vi "Digital Read Pin.vi"(8 "Error In":errorcluster, 10 "Digital I/O Pin (2)":u8=2, 11 "ChipKit Resource":T1={"COM Port"="", "Board Type"=enum."ChipKit uC32", "Connection Type"=enum."USB / Serial", "Baud Rate (115200)"=15, "Bytes Per Packet (15)"=15}) -> (0 "Error Out":errorcluster, 2 "Value":bool, 3 "ChipKit Resource":T1={"COM Port"="", "Board Type"=enum."ChipKit uC32", "Connection Type"=enum."USB / Serial", "Baud Rate (115200)"=15, "Bytes Per Packet (15)"=15})   [LabVIEW 2011, in "LabVIEW Interface for ChipKit.lvlib"]
doc: "Reads the digital value of the selected Arduino digital input pin (D0 - D13). The pin must fist be configured as an input using the Arduino Set Digital Pin Mode VI."
uses:
  LabVIEW Interface for ChipKit.lvlib
  Private/Type Defs/Chipkit Resource.ctl
  Private/Type Defs/Board Type.ctl
  Private/Type Defs/Connection Type.ctl
  Private/Type Defs/Command.ctl
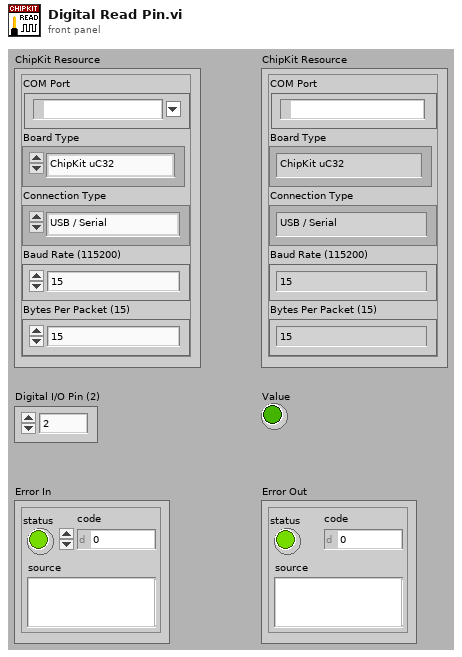
[diagram p1: front panel]
types:
  T1 = typedef "LabVIEW Interface for ChipKit.lvlib/Chipkit Resource.ctl" = cluster{"COM Port":refnum<visa-resource-name>, "Board Type":T2, "Connection Type":T3, "Baud Rate (115200)":u32, "Bytes Per Packet (15)":u32}
  T2 = typedef "LabVIEW Interface for ChipKit.lvlib/Board Type.ctl" = enum16{"ChipKit uC32", "ChipKit Uno32", "ChipKit Max32"}
  T3 = typedef "LabVIEW Interface for ChipKit.lvlib/Connection Type.ctl" = enum8{"USB / Serial", "XBEE", "BlueSmirf (Bluetooth)"}
  T4 = typedef "LabVIEW Interface for ChipKit.lvlib/Command.ctl" = enum8{"setArduinoMode", "flushSerial", "setPinMode", "digitalWritePin", "digitalWritePort", "tone", "digitalReadPin", "digitalReadPort", "analogReadPin", "analogReadPort", "pwmWritePin", "pwmWritePort", "sevenSegment_Configure", "sevenSegment_Write", "I2C Init", "I2C Write", "I2C Read", "SPI Init", "SPI Set Bit Order", "SPI Set Clock Divider", "SPI Set Data Mode", "SPI Send / Receive", "SPI Close", "Servo Set Num Servos", "Servo Config Servo", "Servo Write Angle", "Servo Read Angle", "Servo Write Pulse Width", "Servo Read Pulse Width", "Servo Detach", "LCD Init", "LCD Set Size", "LCD Set Cursor Mode", "LCD Clear", "LCD Set Cursor Position", "LCD Print", "LCD Display Power", "LCD Scroll Display", "LCD Autoscroll", "LCD Print Direction", "LCD Create Custom Char", "LCD Print Custom Char", "contAcqOn", "contAcqOff", "getFirmwareVersion", "FiniteSampleStart"}
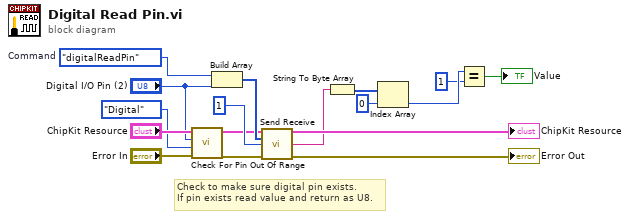
[diagram p0: block diagram]
diagram:
  w17 = Command."digitalReadPin"  # Command
  # "Check to make sure digital pin exists.\nIf pin exists read value and return as U8."
  n1 = call "Check For Pin Out Of Range.vi"("Error In"="Error In", "Pin Type"=enum16{"Analog", "Digital"}."Digital", "User Pin Number"="Digital I/O Pin (2)", "Arduino Resource"="ChipKit Resource") -> ("Error Out"=w10:errorcluster, "Arduino Resource"=w11:T1)  [unwired: 6 in]
  n2 = Build Array(w17, "Digital I/O Pin (2)") -> (w14:u8[])
  n3 = call "Send Receive.vi"("Arduino Resource"=w11, "Data"=w14, "Bytes To Read (0)"=u32 1, "error in"=w10) -> ("Arduino Resource"=→"ChipKit Resource":T1, "Read Buffer"=w7:string, "error out"=→"Error Out":errorcluster)  [unwired: 9 in]
  n4 = String To Byte Array(string=w7) -> (unsigned byte array=w6:u8[])
  n5 = Index Array(array=w6, index=0) -> (element=w3:u8)
  n6 = Equal?(x=w3, y=u8 1) -> (x = y?=→"Value":bool)
